vi "Draw Line.vi"(0 "picture":picture, 2 "end point":cluster{"x":i16, "y":i16}, 3 "absolute coordinates?(T)":bool=TRUE, 4 "color(black)":u32(colorbox), 8 "pen":T1={"Width"=1, "Style"=enum."Solid"}) -> (6 "new picture":picture)   [LabVIEW 2015]
doc: "Draws a line from the current pen position to the specified location in a picture."
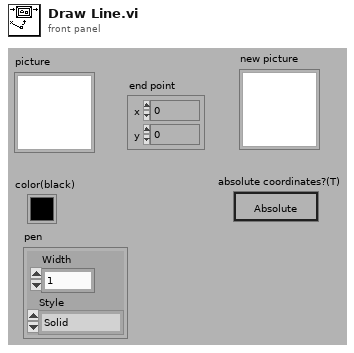
[diagram p1: front panel]
types:
  T1 = cluster{"Width":u16, "Style":enum32{"Solid", "Dash", "Dot", "DashDot", "DashDotDot"}}
  T2 = cluster{"opcode-Line":i16, "size":i32, cluster{"y":i16, "x":i16}}
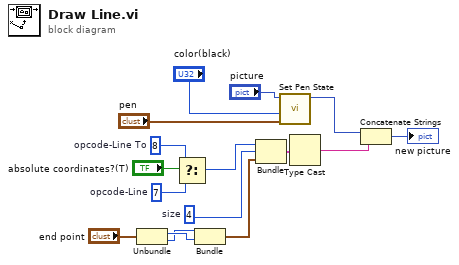
[diagram p0: block diagram]
diagram:
  w14 = i16 7  # opcode-Line
  w15 = i16 8  # opcode-Line To
  w12 = 4  # size
  n1 = Unbundle("end point") -> ("x"=w8:i16, "y"=w7:i16)
  n2 = Select(t=w15, s="absolute coordinates?(T)", f=w14) -> (s? t:f=w13:i16)
  n3 = Bundle("y"=w7, "x"=w8) -> (w6:cluster{"y":i16, "x":i16})  [unwired: 1 in]
  n4 = Bundle("opcode-Line"=w13, "size"=w12, w6) -> (w10:T2)  [unwired: 1 in]
  n5 = call "Set Pen State.vi"("pen"="pen", "color(black)"="color(black)", "Picture"="picture") -> ("Picture 2"=w5:picture)  [unwired: 6 in]
  n6 = Type Cast(x=w10) -> (*(type *) &x=w9:string)  [unwired: 1 in]
  n7 = Concatenate Strings(w5, w9) -> (→"new picture":picture)
